vi "Ver 1.1.vi"() -> ()   [LabVIEW 2016]
doc: "This example VI shows how to use thermocouples to take a temperature measurement.\n\nNote:\nFor front panel measurements, make sure the Input switch is in the out position(F)\nFor plug-in card measurements, make sure the Input switch is in the in poisition(R)"
uses:
  Documents/keithley_27xx/Keithley 27XX/Public/Configure/Measurement Specific/Configure FRTD.vi
  Documents/keithley_27xx/Keithley 27XX/Public/Configure/Measurement Specific/Configure Thermocouple.vi
  Documents/keithley_27xx/Keithley 27XX/Public/Configure/Measurement Specific/Configure Thermistor.vi
  Documents/keithley_27xx/Keithley 27XX/Public/Data/Read Multiple Direct.vi
  Documents/keithley_27xx/Keithley 27XX/Keithley 27XX.lvlib
  Documents/keithley_27xx/Keithley 27XX/Public/Close.vi
panel:
  in  "Sample size":dbl
  in  "Channel (101) 3":string="113"
  out "Output1 3":dbl[](array[numeric])
  in  "Alpha1 3":dbl=0.0038
  in  "Beta1 3":dbl=0.1
  in  "Delta1 3":dbl=1.0
  in  "Sensor Type 3":string(combo)
  in  "Channel (101) 2":string="113"
  out "Output1 2":dbl[](array[numeric])
  in  "Alpha1 2":dbl=0.0038
  in  "Beta1 2":dbl=0.1
  in  "Delta1 2":dbl=1.0
  in  "Sensor Type 2":string(combo)
  in  "Sensor Type":string(combo)
  in  "Delta1":dbl=1.0
  in  "Beta1":dbl=0.1
  in  "Alpha1":dbl=0.0038
  in  "Serial Configuration":T1={"Baud Rate (9600)"=9600, "Flow Control (1: XON/XOFF)"=1, "Termination Char (0:CR)"=0} {"Termination Char (0:CR)" items=["CR", "LF", "CRLF (Do not use)", "LFCR (Do not use)"]; "Flow Control (1: XON/XOFF)" items=["None", "XON/XOFF", "RTS/CTS (2701 Only)", "XON/XOFF & RTS/CTS (2701 Only)"]; "Baud Rate (9600)" items=["300"=300, "600"=600, "1200"=1200, "2400"=2400, "4800"=4800, "9600"=9600, "19.2k"=19200, "38.4k (2701 Only)"=38400, "57.6k (2701 Only)"=57600, "115.2k (2701 Only)"=115200]}
  in  "VISA resource name":refnum<visa-resource-name>="TCPIP0::192.168.69.200::1394::SOCKET"
  in  "stop":bool
  out "Output1":dbl[](array[numeric])
  in  "Channel (101)":string="113"
  in  "Temperature (0: Celsius)":u16(ring) items=["Celsius", "Fahrenheit", "Kelvin"]
  # "*For front panel measurements, make sure the Input switch is in the out position(F)*\n  For plug-in card measurements, make sure the Input switch is in the in position(R)"
  # "© 2005 National Instruments Corporation.  ALL RIGHTS RESERVED."
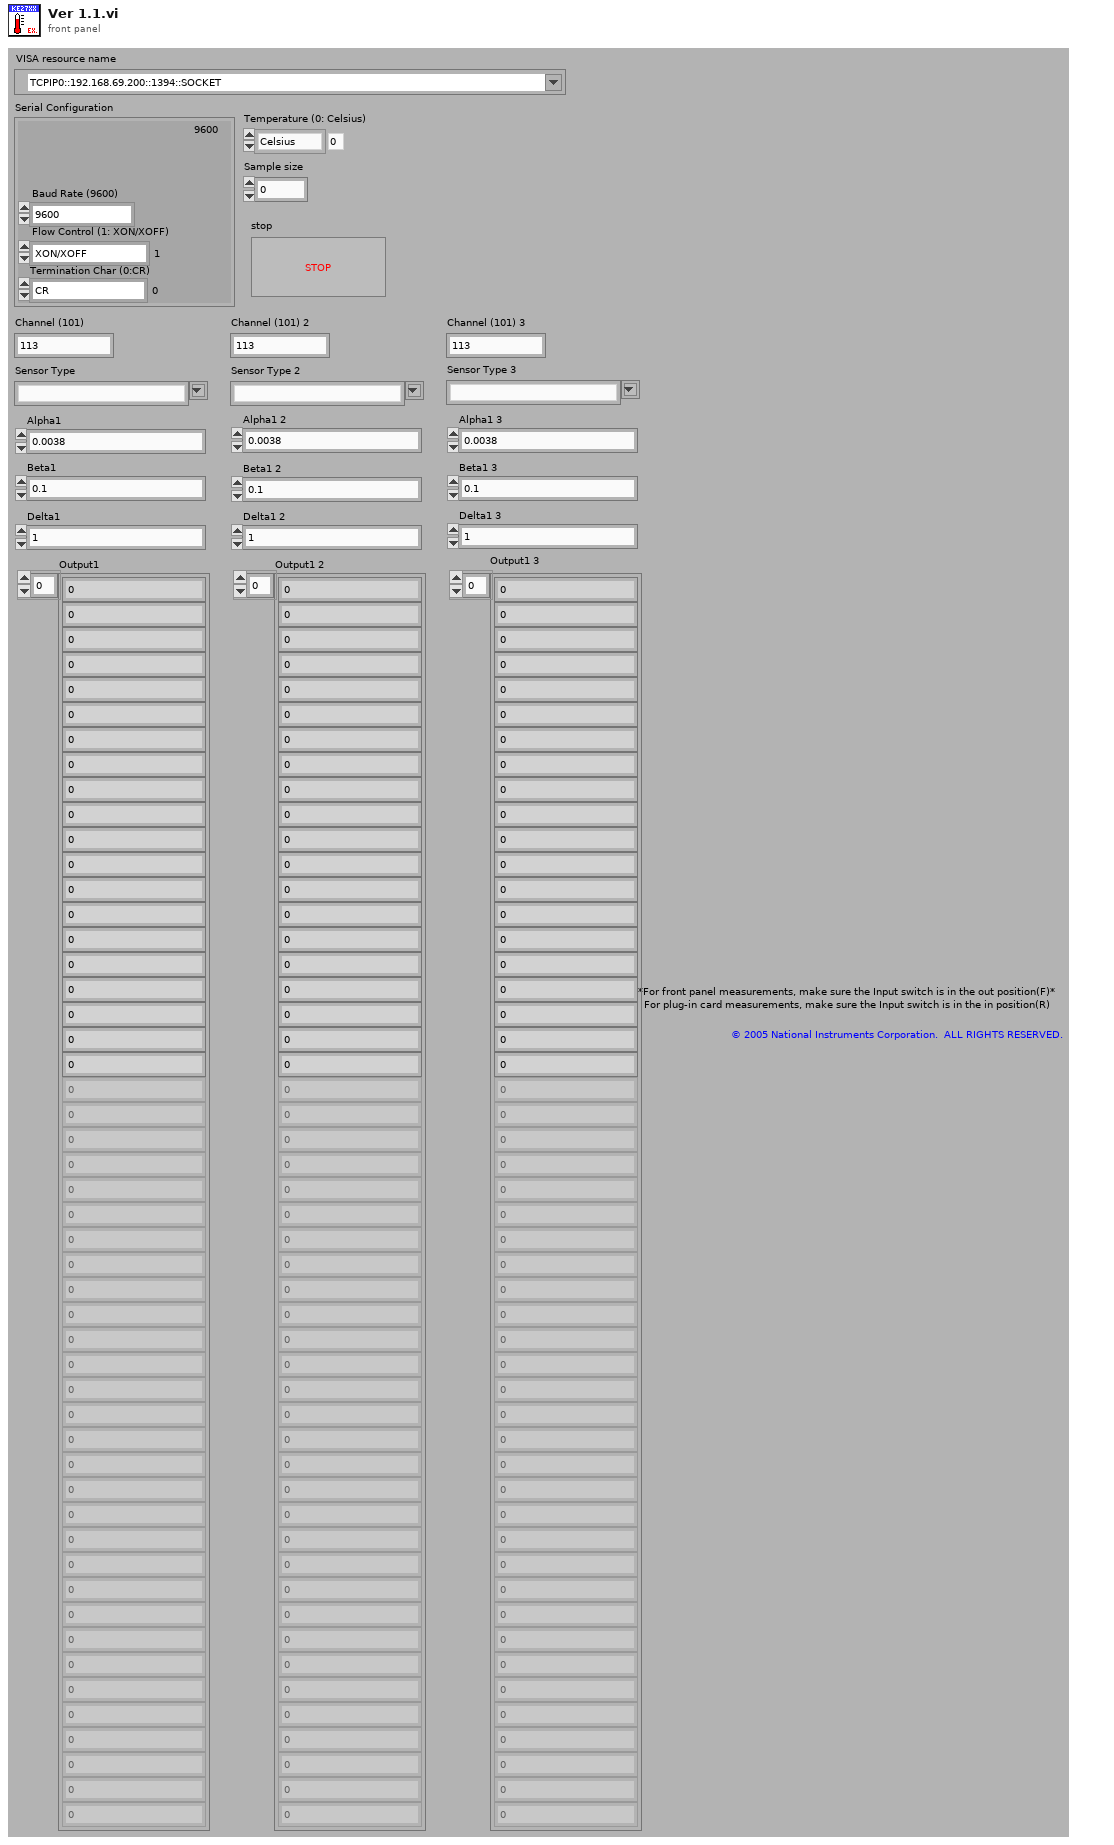
[diagram p1: front panel]
types:
  T1 = cluster{"Baud Rate (9600)":u32, "Flow Control (1: XON/XOFF)":u16, "Termination Char (0:CR)":u16}
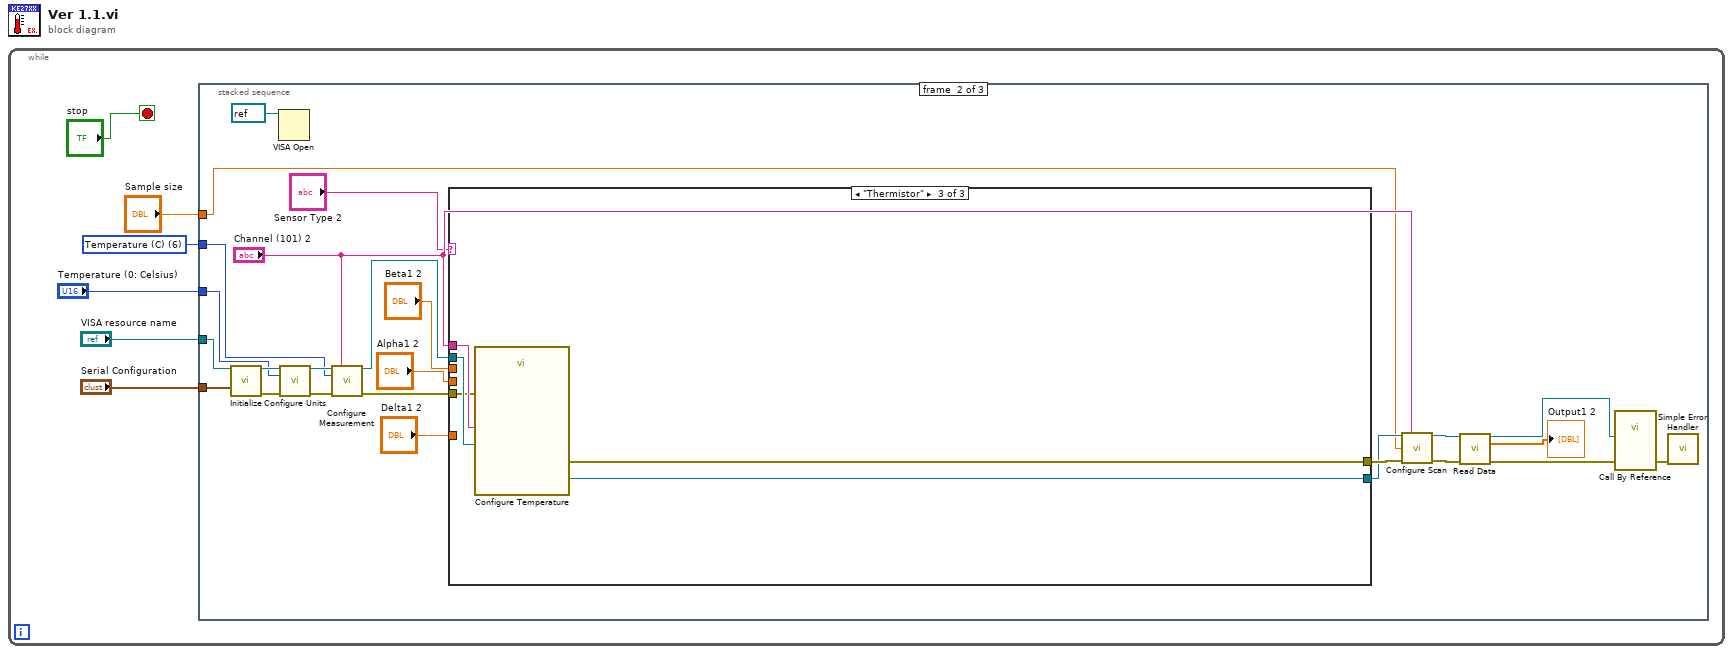
[diagram p0: block diagram]
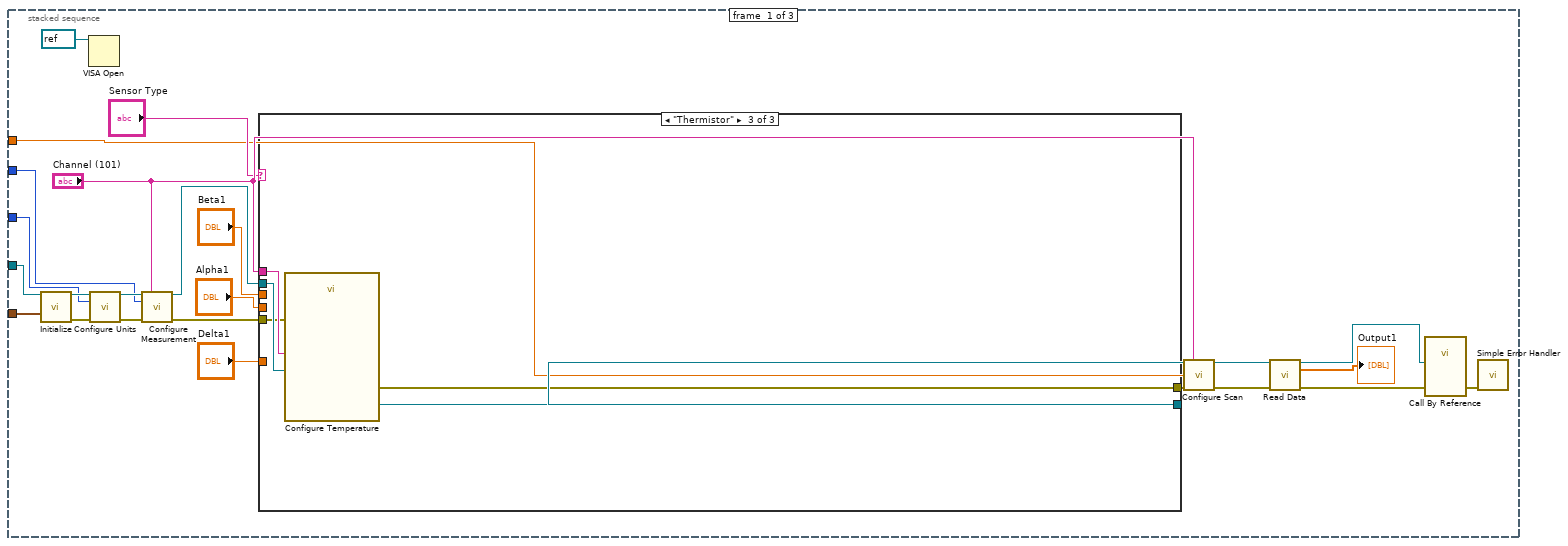
[diagram p2: hidden frame]
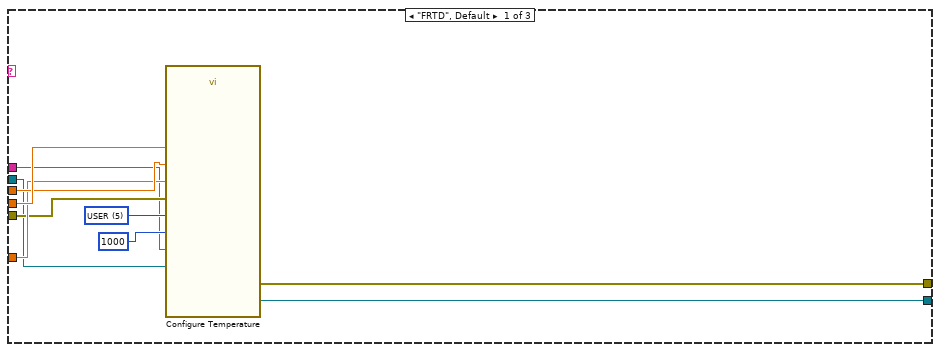
[diagram p3: hidden frame]
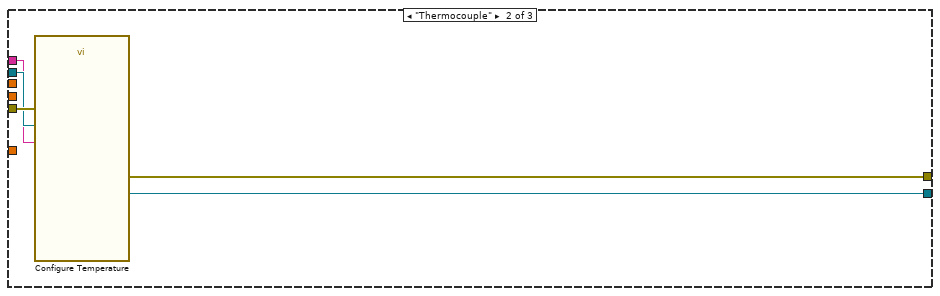
[diagram p4: hidden frame]
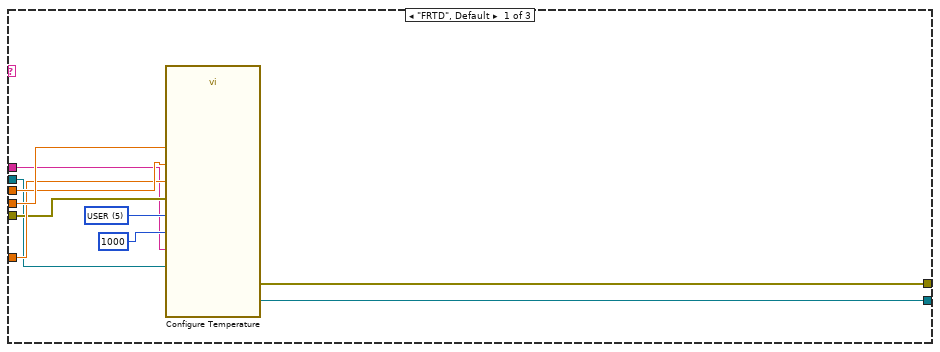
[diagram p5: hidden frame]
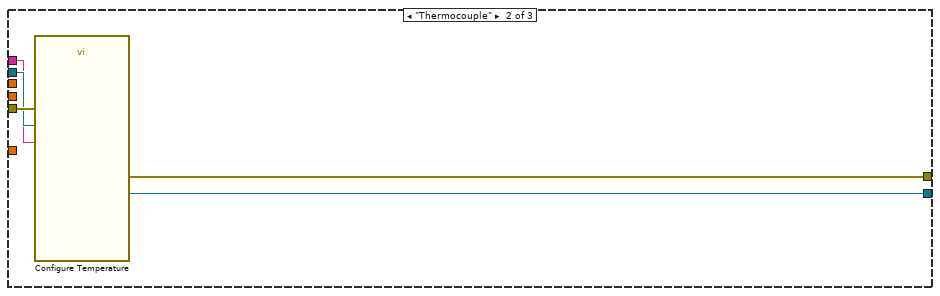
[diagram p6: hidden frame]
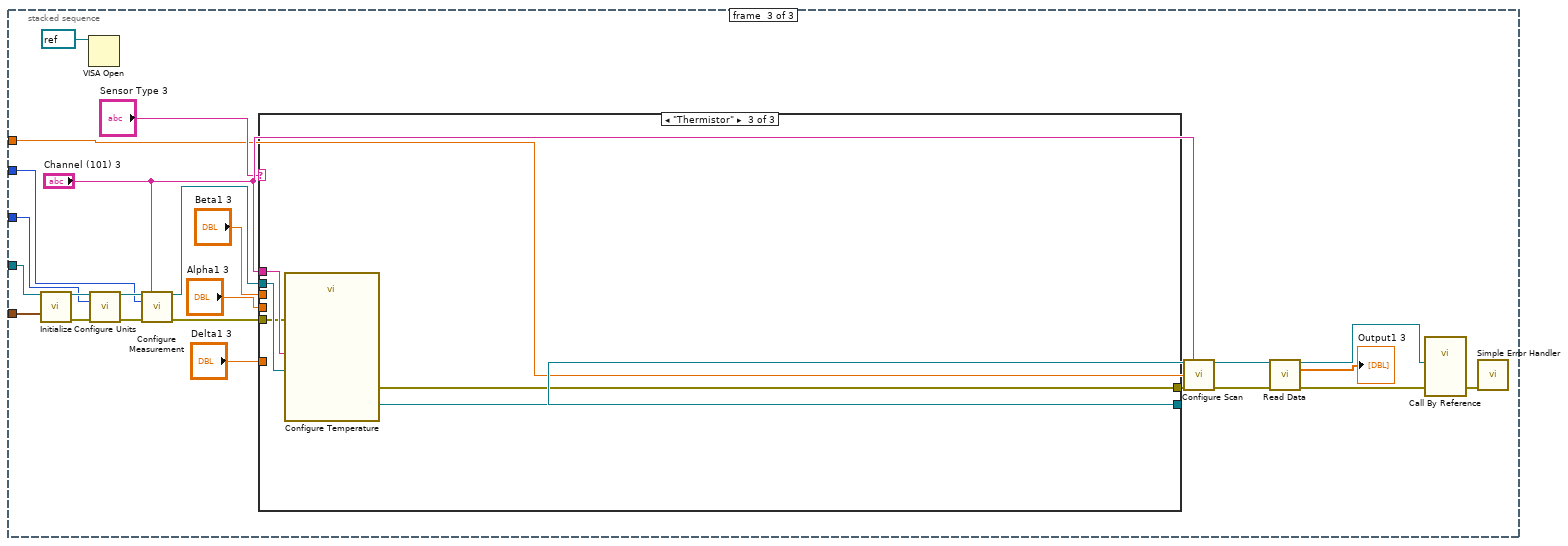
[diagram p7: hidden frame]
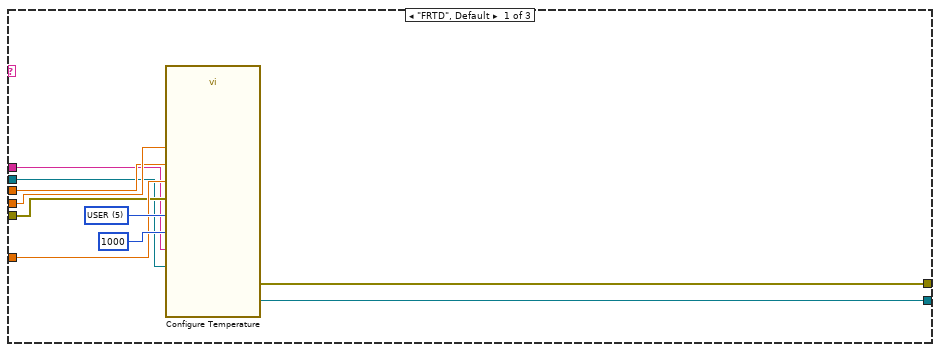
[diagram p8: hidden frame]
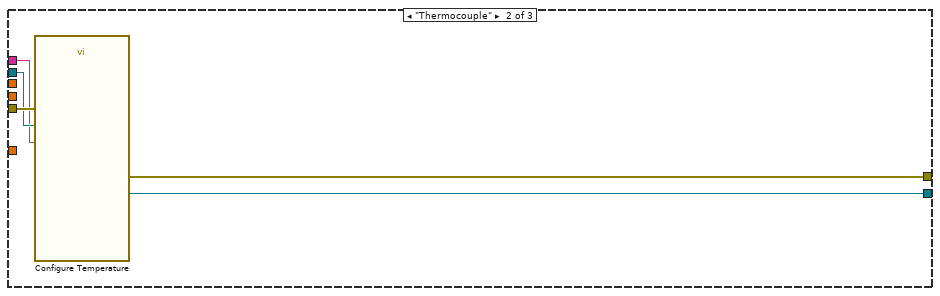
[diagram p9: hidden frame]
diagram:
  n1 = while {
    stop <- "stop" stop-if-true
    w4 = u16 6 items=["DC Voltage", "AC Voltage", "DC Current", "AC Current", "Resistance", "Four-Wire Resistance", "Temperature (C)", "Frequency", "Period", "Continuity"] ("Function (0: DC Voltage)")
    n2 = stacked-sequence {
      tunnel: "VISA resource name" -> [w23 w68 w113]
      tunnel: "Serial Configuration" -> [w22 w67 w112]
      tunnel: w4 -> [w21 w66 w111]
      tunnel: "Temperature (0: Celsius)" -> [w20 w65 w110]
      tunnel: "Sample size" -> [w8 w53 w98]
      frame #0 {
        n3 = call "Initialize.vi"("VISA resource name"=w23, "Serial Configuration"=w22) -> ("VISA resource name out"=w30:refnum<visa-resource-name>, "error out"=w27:errorcluster)  [unwired: 12 in]
        n4 = VISA Open(VISA resource name=refnum<visa-resource-name> refnum) -> ()  [unwired: 4 in, 2 out]
        n5 = call "Configure Units.vi"("VISA resource name"=w30, "Temperature (0: Celsius)"=w20, "error in (no error)"=w27) -> ("VISA resource name out"=w31:refnum<visa-resource-name>, "error out"=w26:errorcluster)  [unwired: 11 in]
        n6 = call "Configure Measurement.vi"("VISA resource name"=w31, "Scan List (Empty)"="Channel (101)", "Function (0: DC Voltage)"=w21, "error in (no error)"=w26) -> ("VISA resource name out"=w13:refnum<visa-resource-name>, "error out"=w14:errorcluster)  [unwired: 10 in]
        n7 = case shown="\"Thermistor\"" "Sensor Type" {
          tunnel: [w40 w45 w51] -> w19
          tunnel: [w41 w46 w50] -> w18
          tunnel: "Delta1" -> [w35 _ _]
          tunnel: "Beta1" -> [w36 _ _]
          tunnel: "Alpha1" -> [w37 _ _]
          tunnel: w14 -> [w34 w44 w47]
          tunnel: w13 -> [w33 w43 w48]
          tunnel: "Channel (101)" -> [w32 w42 w49]
          frame "FRTD", Default {
            w39 = u16 5 items=["PT100", "D100", "F100", "PT3916", "PT385", "USER"] ("FRTD Type (0: PT100)")
            n8 = call-poly "Configure Temperature.vi"("VISA resource name"=w33, "FRTD Type (0: PT100)"=w39, "error in (no error)"=w34, "Scan List (Empty)"=w32, "R Zero (100)"=1000, "Alpha (0.00385)"=w37, "Beta (0.111)"=w36, "Delta (1.507)"=w35) -> ("VISA resource name out"=w41:refnum<visa-resource-name>, "error out"=w40:errorcluster)  [unwired: 10 in]
          }
          frame "Thermocouple" {
            n9 = call-poly "Configure Temperature.vi"("VISA resource name"=w43, "error in (no error)"=w44, "Scan List (Empty)"=w42) -> ("VISA resource name out"=w46:refnum<visa-resource-name>, "error out"=w45:errorcluster)  [unwired: 15 in]
          }
          frame "Thermistor" {
            n10 = call-poly "Configure Temperature.vi"("VISA resource name"=w48, "error in (no error)"=w47, "Scan List (Empty)"=w49) -> ("VISA resource name out"=w50:refnum<visa-resource-name>, "error out"=w51:errorcluster)  [unwired: 15 in]
          }
        }
        n11 = call "Configure Scan.vi"("VISA resource name"=w18, "Channel List (101:110)"="Channel (101)", "Sample Count (100)"=w8, "error in (no error)"=w19) -> ("VISA resource name out"=w28:refnum<visa-resource-name>, "error out"=w29:errorcluster)  [unwired: 10 in]
        n12 = call-poly "Read Data.vi"("VISA resource name"=w28, "error in (no error)"=w29) -> ("VISA resource name out"=w9:refnum<visa-resource-name>, "Measurement Data"=→"Output1":dbl[], "error out"=w10:errorcluster)  [unwired: 8 in, 3 out]
        n13 = call-by-ref "?"("VISA resource name"=w9, "error in (no error)"=w10) -> ("error out"=w7:errorcluster)  [unwired: 15 in, 2 out]
        n14 = call <vilib>:"Simple Error Handler.vi"("error in (no error)"=w7) -> ()  [unwired: 4 in, 5 out]
      }
      frame #1 {
        n15 = call "Initialize.vi"("VISA resource name"=w68, "Serial Configuration"=w67) -> ("VISA resource name out"=w75:refnum<visa-resource-name>, "error out"=w72:errorcluster)  [unwired: 12 in]
        n16 = VISA Open(VISA resource name=refnum<visa-resource-name> refnum) -> ()  [unwired: 4 in, 2 out]
        n17 = call "Configure Units.vi"("VISA resource name"=w75, "Temperature (0: Celsius)"=w65, "error in (no error)"=w72) -> ("VISA resource name out"=w76:refnum<visa-resource-name>, "error out"=w71:errorcluster)  [unwired: 11 in]
        n18 = call "Configure Measurement.vi"("VISA resource name"=w76, "Scan List (Empty)"="Channel (101) 2", "Function (0: DC Voltage)"=w66, "error in (no error)"=w71) -> ("VISA resource name out"=w58:refnum<visa-resource-name>, "error out"=w59:errorcluster)  [unwired: 10 in]
        n19 = case shown="\"Thermistor\"" "Sensor Type 2" {
          tunnel: [w85 w90 w96] -> w64
          tunnel: [w86 w91 w95] -> w63
          tunnel: "Delta1 2" -> [w80 _ _]
          tunnel: "Beta1 2" -> [w81 _ _]
          tunnel: "Alpha1 2" -> [w82 _ _]
          tunnel: w59 -> [w79 w89 w92]
          tunnel: w58 -> [w78 w88 w93]
          tunnel: "Channel (101) 2" -> [w77 w87 w94]
          frame "FRTD", Default {
            w84 = u16 5 items=["PT100", "D100", "F100", "PT3916", "PT385", "USER"] ("FRTD Type (0: PT100)")
            n20 = call-poly "Configure Temperature.vi"("VISA resource name"=w78, "FRTD Type (0: PT100)"=w84, "error in (no error)"=w79, "Scan List (Empty)"=w77, "R Zero (100)"=1000, "Alpha (0.00385)"=w82, "Beta (0.111)"=w81, "Delta (1.507)"=w80) -> ("VISA resource name out"=w86:refnum<visa-resource-name>, "error out"=w85:errorcluster)  [unwired: 10 in]
          }
          frame "Thermocouple" {
            n21 = call-poly "Configure Temperature.vi"("VISA resource name"=w88, "error in (no error)"=w89, "Scan List (Empty)"=w87) -> ("VISA resource name out"=w91:refnum<visa-resource-name>, "error out"=w90:errorcluster)  [unwired: 15 in]
          }
          frame "Thermistor" {
            n22 = call-poly "Configure Temperature.vi"("VISA resource name"=w93, "error in (no error)"=w92, "Scan List (Empty)"=w94) -> ("VISA resource name out"=w95:refnum<visa-resource-name>, "error out"=w96:errorcluster)  [unwired: 15 in]
          }
        }
        n23 = call "Configure Scan.vi"("VISA resource name"=w63, "Channel List (101:110)"="Channel (101) 2", "Sample Count (100)"=w53, "error in (no error)"=w64) -> ("VISA resource name out"=w73:refnum<visa-resource-name>, "error out"=w74:errorcluster)  [unwired: 10 in]
        n24 = call-poly "Read Data.vi"("VISA resource name"=w73, "error in (no error)"=w74) -> ("VISA resource name out"=w54:refnum<visa-resource-name>, "Measurement Data"=→"Output1 2":dbl[], "error out"=w55:errorcluster)  [unwired: 8 in, 3 out]
        n25 = call-by-ref "?"("VISA resource name"=w54, "error in (no error)"=w55) -> ("error out"=w52:errorcluster)  [unwired: 15 in, 2 out]
        n26 = call <vilib>:"Simple Error Handler.vi"("error in (no error)"=w52) -> ()  [unwired: 4 in, 5 out]
      }
      frame #2 {
        n27 = call "Initialize.vi"("VISA resource name"=w113, "Serial Configuration"=w112) -> ("VISA resource name out"=w120:refnum<visa-resource-name>, "error out"=w117:errorcluster)  [unwired: 12 in]
        n28 = VISA Open(VISA resource name=refnum<visa-resource-name> refnum) -> ()  [unwired: 4 in, 2 out]
        n29 = call "Configure Units.vi"("VISA resource name"=w120, "Temperature (0: Celsius)"=w110, "error in (no error)"=w117) -> ("VISA resource name out"=w121:refnum<visa-resource-name>, "error out"=w116:errorcluster)  [unwired: 11 in]
        n30 = call "Configure Measurement.vi"("VISA resource name"=w121, "Scan List (Empty)"="Channel (101) 3", "Function (0: DC Voltage)"=w111, "error in (no error)"=w116) -> ("VISA resource name out"=w103:refnum<visa-resource-name>, "error out"=w104:errorcluster)  [unwired: 10 in]
        n31 = case shown="\"Thermistor\"" "Sensor Type 3" {
          tunnel: [w130 w135 w141] -> w109
          tunnel: [w131 w136 w140] -> w108
          tunnel: "Delta1 3" -> [w125 _ _]
          tunnel: "Beta1 3" -> [w126 _ _]
          tunnel: "Alpha1 3" -> [w127 _ _]
          tunnel: w104 -> [w124 w134 w137]
          tunnel: w103 -> [w123 w133 w138]
          tunnel: "Channel (101) 3" -> [w122 w132 w139]
          frame "FRTD", Default {
            w129 = u16 5 items=["PT100", "D100", "F100", "PT3916", "PT385", "USER"] ("FRTD Type (0: PT100)")
            n32 = call-poly "Configure Temperature.vi"("VISA resource name"=w123, "FRTD Type (0: PT100)"=w129, "error in (no error)"=w124, "Scan List (Empty)"=w122, "R Zero (100)"=1000, "Alpha (0.00385)"=w127, "Beta (0.111)"=w126, "Delta (1.507)"=w125) -> ("VISA resource name out"=w131:refnum<visa-resource-name>, "error out"=w130:errorcluster)  [unwired: 10 in]
          }
          frame "Thermocouple" {
            n33 = call-poly "Configure Temperature.vi"("VISA resource name"=w133, "error in (no error)"=w134, "Scan List (Empty)"=w132) -> ("VISA resource name out"=w136:refnum<visa-resource-name>, "error out"=w135:errorcluster)  [unwired: 15 in]
          }
          frame "Thermistor" {
            n34 = call-poly "Configure Temperature.vi"("VISA resource name"=w138, "error in (no error)"=w137, "Scan List (Empty)"=w139) -> ("VISA resource name out"=w140:refnum<visa-resource-name>, "error out"=w141:errorcluster)  [unwired: 15 in]
          }
        }
        n35 = call "Configure Scan.vi"("VISA resource name"=w108, "Channel List (101:110)"="Channel (101) 3", "Sample Count (100)"=w98, "error in (no error)"=w109) -> ("VISA resource name out"=w118:refnum<visa-resource-name>, "error out"=w119:errorcluster)  [unwired: 10 in]
        n36 = call-poly "Read Data.vi"("VISA resource name"=w118, "error in (no error)"=w119) -> ("VISA resource name out"=w99:refnum<visa-resource-name>, "Measurement Data"=→"Output1 3":dbl[], "error out"=w100:errorcluster)  [unwired: 8 in, 3 out]
        n37 = call-by-ref "?"("VISA resource name"=w99, "error in (no error)"=w100) -> ("error out"=w97:errorcluster)  [unwired: 15 in, 2 out]
        n38 = call <vilib>:"Simple Error Handler.vi"("error in (no error)"=w97) -> ()  [unwired: 4 in, 5 out]
      }
    }
  }
